vi "Subvi Boolean Stretcher Copy3.vi"(0 "Bool Refnum":refnum<vi>, 1 "Trigger":bool, 2 "Delay Cycles":u32=10) -> ()   [LabVIEW 2012]
panel:
  out "Stretched":bool
  out "stop":bool
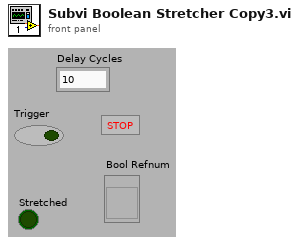
[diagram p1: front panel]
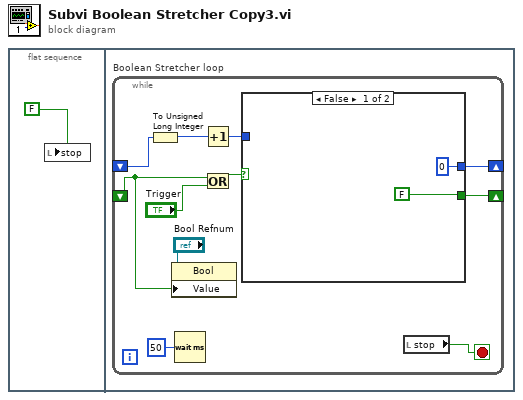
[diagram p0: block diagram]
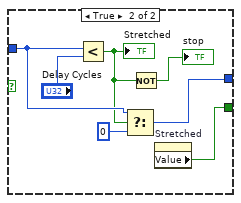
[diagram p2: hidden frame]
diagram:
  n1 = flat-sequence {
    frame #0 {
      n2 = local write "stop"(FALSE) -> ()
    }
    frame #1 {
      n3 = while "Boolean Stretcher loop" {
        shift-right: [w11] -> _
        shift-left: _ -> [w3]
        shift-right: [w9] -> _
        shift-left: _ -> [w2]
        stop <- w5 stop-if-true
        n4 = To Unsigned Long Integer(number=w3) -> (unsigned 32bit integer=w10:u32)
        n5 = property class="Bool"(reference="Bool Refnum", "Value"=w2) -> ()  [unwired: 1 in, 2 out]
        n6 = Wait (ms)(milliseconds to wait=u32 50) -> ()  [unwired: 1 out]
        n7 = Increment(x=w10) -> (x+1=w12:u32)
        n8 = Or(x=w2, y="Trigger") -> (x .or. y?=w7:bool)
        n9 = case shown="False" w7 {
          tunnel: w12 -> [_ w21]
          tunnel: [FALSE w18] -> w9
          tunnel: [u32 0 ("f") w19] -> w11
          frame False {
          }
          frame True {
            n10 = Less?(x=w21, y="Delay Cycles") -> (x < y?=w15:bool)
            "Stretched" <- w15
            n11 = Select(t=w21, s=w15, f=u32 0) -> (s? t:f=w19:u32)
            n12 = Not(x=w15) -> (.not. x?=→"stop":bool)
            n13 = property on="Stretched" class="Bool (strict)"() -> ("Value"=w18:bool)  [unwired: 2 in, 2 out]
          }
        }
        n14 = local read "stop"() -> (w5:bool)
      }
    }
  }
